vi "onCreate.vi"(8 "error in (no error)":errorcluster, 11 "PolyA":refnum<class "PolyA.lvclass">) -> (0 "error out":errorcluster, 3 "PolyA out":refnum<class "PolyA.lvclass">)   [LabVIEW 2014, in "PolyA.lvclass"]
doc: "JKI State Machine Objects (SMO) 1.4.0.57\nJKI - JKI\nCopyright (c) 2018, JKI"
uses:
  PolyA.lvclass
  Query Payload -- cluster.ctl
  PolyA.lvclass/PolyA.ctl
  <vilib>/JKI/JKI SMO/SMO/SMO.lvclass
panel:
  # "For instructions on how to use the JKI State Machine Objects, examples and video tutorials, visit:\nhttp://jki.net/state-machine-objects/\n\nJKI State Machine Objects™\nhttp://jki.net/state-machine-objects/\nCopyright (C) 2005-2015, JKI <info@jki.net>\nALL RIGHTS RESERVED"
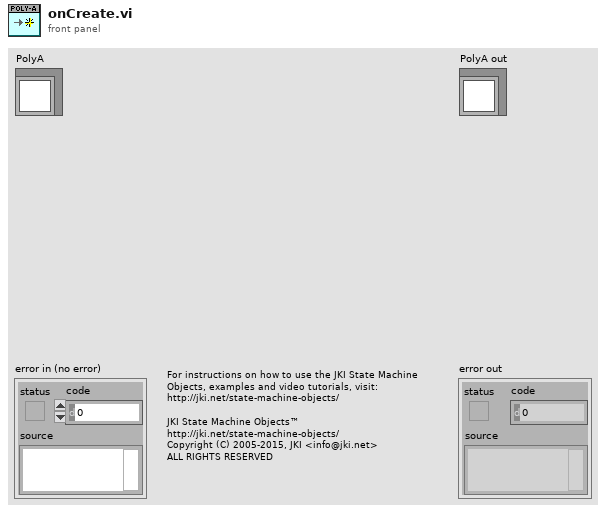
[diagram p1: front panel]
types:
  T1 = typedef "PolyA.lvclass/Query Payload -- cluster.ctl" = cluster{"value":dbl, "notifier":refnum<notifier>}
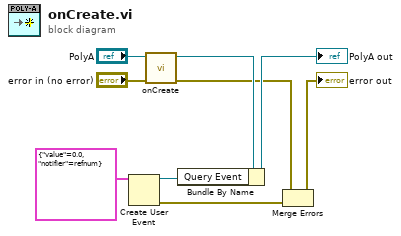
[diagram p0: block diagram]
diagram:
  n1 = Create User Event(user event datatype=T1 {"value"=0.0, "notifier"=refnum} ("Query Payload")) -> (user event=w2:refnum<user-event>, error out=w1:errorcluster)  [unwired: 1 in]
  n2 = call-parent "onCreate.vi"("error in (no error)"="error in (no error)", "SMO"="PolyA") -> ("error out"=w5:errorcluster, "SMO out"=w9:refnum<class "PolyA.lvclass">)  [unwired: 8 in]
  n3 = Bundle By Name(cluster=w9, "Query Event"=w2) -> (→"PolyA out":refnum<class "PolyA.lvclass">)
  n4 = Merge Errors(w5, w1) -> (→"error out":errorcluster)
